vi "Library.Save.vi"(8 "error in (no error)":errorcluster, 10 "Path":path, 11 "Library Reference":refnum<vi>) -> (0 "error out":errorcluster, 3 "dup Library Reference":refnum<vi>)   [LabVIEW 2011]
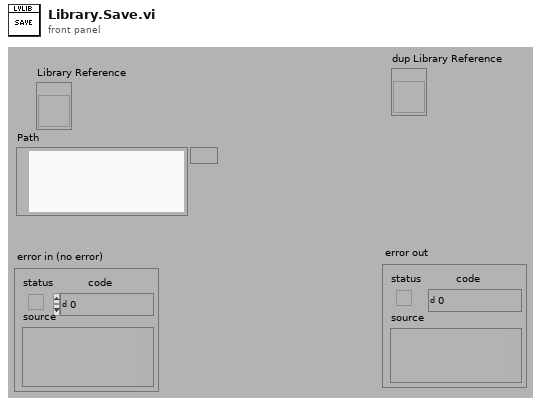
[diagram p1: front panel]
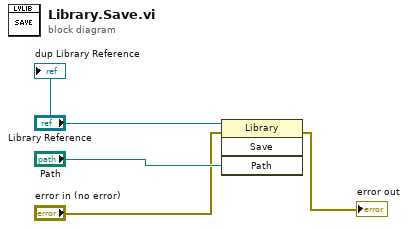
[diagram p0: block diagram]
diagram:
  n1 = invoke class="Library" method="Save"(reference="Library Reference", error in="error in (no error)", "Path"="Path") -> (error out=→"error out":errorcluster)  [unwired: 1 in, 3 out]
  "dup Library Reference" <- "Library Reference"
